vi "test_Create MetaData Channel_error on name collision.vi"(8 "error in (no error)":errorcluster, 11 "TestCase in":refnum<class "Instrument Addon Scripting API Channels Unit Tests.lvclass">) -> (0 "error out":errorcluster, 3 "TestCase out":refnum<class "Instrument Addon Scripting API Channels Unit Tests.lvclass">)   [LabVIEW 2019, in "Instrument Addon Scripting API Channels Unit Tests.lvclass"]
uses:
  Instrument Addon Scripting API Channels Unit Tests.lvclass
  APIs/Scripting API/TypeDefs/Single Channel Type Cast Settings.ctl
  Addon/Addon Shared/Types/Type Cast Type.ctl
  Addon/Addon Shared/Types/Endian.ctl
  APIs/Scripting API/TypeDefs/Single Channel Format Settings.ctl
  Instrument Addon Scripting API Channels Unit Tests.lvclass/Instrument Addon Scripting API Channels Unit Tests.ctl
  <vilib>/NI VeriStand/Custom Device Tools/Custom Device Utility Library/NI VeriStand - Search for Item by Name.vi
  APIs/Scripting API/Channels/Create MetaData Channel - Single Channel - Type Cast.vi
  APIs/Scripting API/Channels/Create MetaData Channel - Single Channel - Format.vi
  <vilib>/addons/_JKI Toolkits/VI Tester/TestCase.llb/TestCase.lvclass
  <vilib>/NI VeriStand/Custom Device Tools/Custom Device Utility Library/Custom Device Utility Library.lvlib
  Addon/Addon Shared/Instrument Addon Shared.lvlib
  APIs/Scripting API/Instrument Addon Scripting API.lvlib
  C:/Program Files (x86)/National Instruments/LabVIEW 2019/vi.lib/addons/_JKI Toolkits/VI Tester/TestCase.llb/TestCase.lvclass
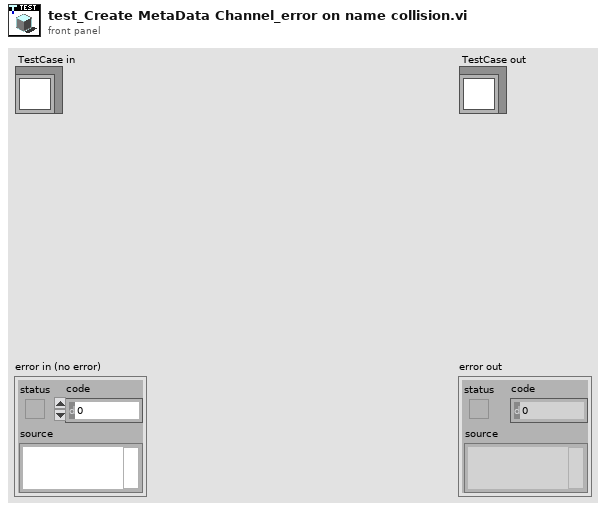
[diagram p1: front panel]
types:
  T1 = typedef "Instrument Addon Scripting API.lvlib/Single Channel Format Settings.ctl" = cluster{"Format String":string, "Default Value":dbl, "Units":string}
  T2 = typedef "Instrument Addon Scripting API.lvlib/Single Channel Type Cast Settings.ctl" = cluster{"Default Value":dbl, "Units":string, "Type":T3, "Endian":T4}
  T3 = typedef "Instrument Addon Shared.lvlib/Type Cast Type.ctl" = enum16{"DBL", "SGL", "U64", "U32", "U16", "U8", "I64", "I32", "I16", "I8"}
  T4 = typedef "Instrument Addon Shared.lvlib/Endian.ctl" = enum16{"Native", "Little", "Big"}
  T5 = typedef "Custom Device API.lvlib/Custom Device Item Ref.ctl" = u64
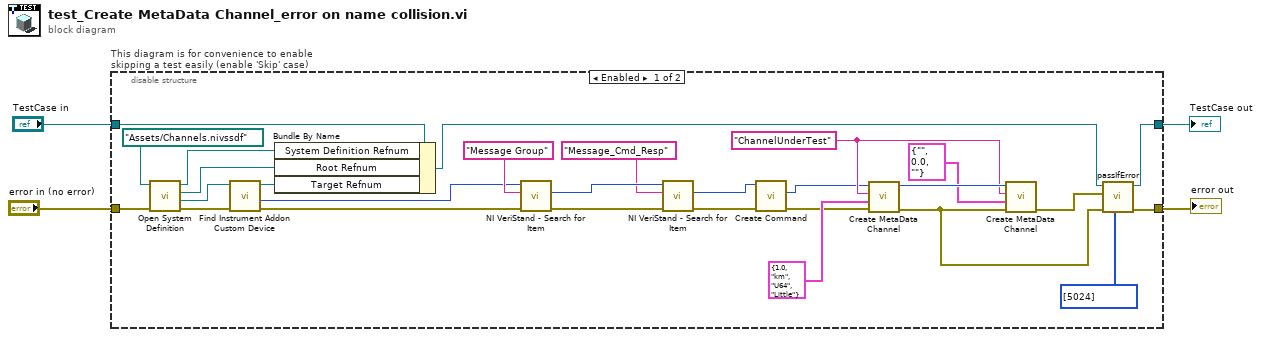
[diagram p0: block diagram]
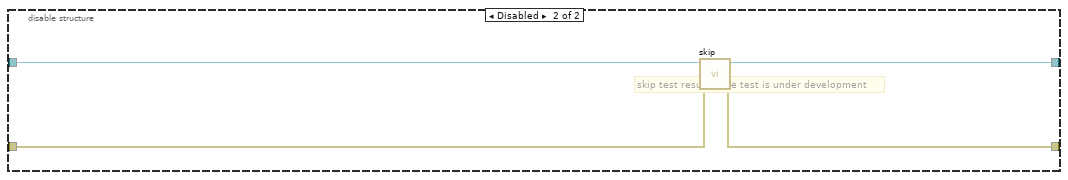
[diagram p2: hidden frame]
diagram:
  n1 = disable-structure "This diagram is for convenience to enable skipping a test easily (enable 'Skip' case)" shown="Enabled" {
    disable-tunnel: "TestCase in" -> [w24 w36]
    disable-tunnel: [w29 w34] -> w1
    disable-tunnel: [w28 w35] -> w3
    disable-tunnel: "error in (no error)" -> [w32 w33]
    frame Enabled {
      w14 = "ChannelUnderTest" ("Name")
      n2 = call "Open System Definition.vi"("error in (no error)"=w32, "System Definition File"=path "Assets/Channels.nivssdf") -> ("error out"=w30:errorcluster, "Target Refnum"=w31:refnum<k24>, "Root Refnum"=w26:refnum<k24>, "System Definition Refnum"=w25:refnum<k24>)  [unwired: 6 in]
      n3 = call "Find Instrument Addon Custom Device.vi"("error in"=w30, "target in"=w31) -> ("error out"=w19:errorcluster, "NodeID"=w18:u64, "target out"=w27:refnum<k24>)  [unwired: 7 in]
      n4 = Bundle By Name(cluster=w24, "System Definition Refnum"=w25, "Root Refnum"=w26, "Target Refnum"=w27) -> (w16:refnum<class "Instrument Addon Scripting API Channels Unit Tests.lvclass">)
      n5 = call-poly <vilib>:"NI VeriStand - Search for Item.vi"("error in"=w19, "Item Name"="Message Group", "Section Ref in"=w18) -> ("error out"=w20:errorcluster, "Item Ref"=w22:T5)  [unwired: 5 in, 2 out]
      n6 = call-poly <vilib>:"NI VeriStand - Search for Item.vi"("error in"=w20, "Item Name"="Message_Cmd_Resp", "Section Ref in"=w22) -> ("error out"=w8:errorcluster, "Item Ref"=w6:T5)  [unwired: 5 in, 2 out]
      n7 = call "Create Command.vi"("error in"=w8, "message refnum In"=w6) -> ("error out"=w7:errorcluster, "command refnum"=w5:T5)  [unwired: 7 in, 1 out]
      n8 = call-poly "Create MetaData Channel.vi"("error in (no error)"=w7, "settings"=T2 {"Default Value"=1.0, "Units"="km", "Type"=enum."U64", "Endian"=enum."Little"} ("Settings"), "channel name"=w14, "command refnum in"=w5) -> ("error out"=w10:errorcluster, "command refnum out"=w15:T5)  [unwired: 5 in, 1 out]
      n9 = call-poly "Create MetaData Channel.vi"("error in (no error)"=w10, "settings"=T1 {"Format String"="", "Default Value"=0.0, "Units"=""} ("Settings"), "channel name"=w14, "command refnum in"=w15) -> ("error out"=w11:errorcluster)  [unwired: 5 in, 2 out]
      n10 = call-dynamic "passIfError.vi"("passing error codes (default = any error code)"=i32[] [5024], "error in (no error)"=w10, "error"=w11, "TestCase in"=w16) -> ("error out"=w28:errorcluster, "TestCase out"=w29:refnum<class "Instrument Addon Scripting API Channels Unit Tests.lvclass">)  [unwired: 6 in]
    }
    frame Disabled {
      # "skip test result while test is under development"
      n11 = call <vilib>:"skip.vi"("error in (no error)"=w33, "TestCase in"=w36) -> ("error out"=w35:errorcluster, "TestCase out"=w34:refnum<class "Instrument Addon Scripting API Channels Unit Tests.lvclass">)  [unwired: 8 in]
    }
  }
  "error out" <- w3
  "TestCase out" <- w1
